vi "ard2.vi"() -> ()   [LabVIEW 2020]
uses:
  <vilib>/Instr/_visa.llb/VISA Configure Serial Port (Instr).vi
panel:
  in  "string":string
  out "concatenated string 2":string
  in  "Boolean 2":bool
  in  "VISA resource name":refnum<visa-resource-name>
  in  "Boolean":bool
  in  "stop":bool
  out "concatenated string":string
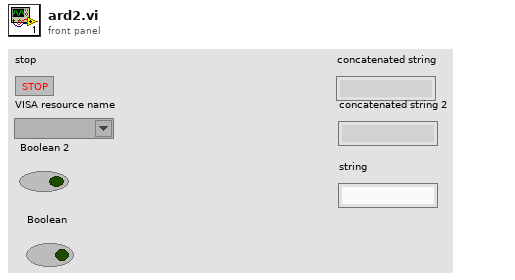
[diagram p1: front panel]
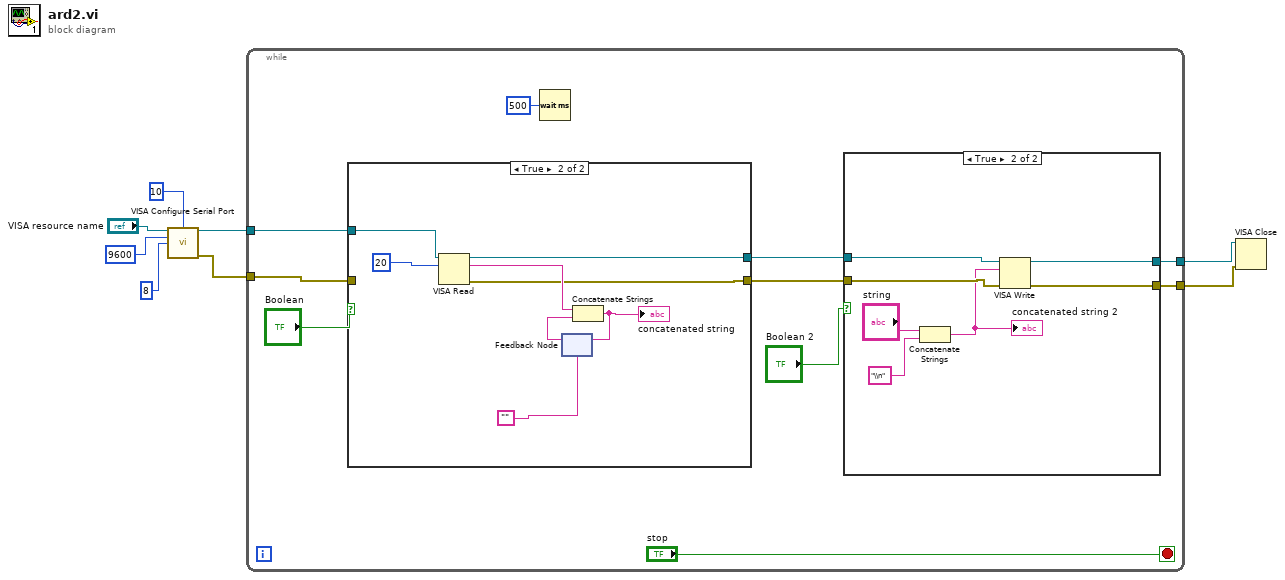
[diagram p0: block diagram]
diagram:
  n1 = call-poly "VISA Configure Serial Port"("VISA resource name"="VISA resource name", "termination char\n(0xA = '\\n' = LF)"=u8 10 ("termination char\n(0xA = '\\n' = LF)"), "baud rate (9600)"=u32 9600, "data bits (8)"=u16 8) -> ("VISA resource name out"=w8:refnum<visa-resource-name>, "error out"=w7:errorcluster)  [unwired: 10 in]
  n2 = while {
    tunnel: w8 -> [w17]
    tunnel: w7 -> [w16]
    tunnel: [w10] -> w2
    tunnel: [w9] -> w1
    stop <- "stop" stop-if-true
    n3 = case shown="True" "Boolean" {
      tunnel: [w28 w31] -> w13
      tunnel: [w29 w33] -> w12
      tunnel: w17 -> [w29 w32]
      tunnel: w16 -> [w28 _]
      frame False {
      }
      frame True {
        n4 = VISA Read(VISA resource name=w32, byte count=u32 20) -> (VISA resource name out=w33:refnum<visa-resource-name>, read buffer=w36:string, error out=w31:errorcluster)  [unwired: 1 in, 1 out]
        n5 = feedback #1("") -> (w34:string)
        n6 = Concatenate Strings(w36, w34) -> (w35:string)
        "concatenated string" <- w35
        n7 = feedback-in #1(w35) -> ()
      }
    }
    n8 = Wait (ms)(milliseconds to wait=u32 500) -> ()  [unwired: 1 out]
    n9 = case shown="True" "Boolean 2" {
      tunnel: w13 -> [w19 w26]
      tunnel: w12 -> [w20 w27]
      tunnel: [w20 w22] -> w10
      tunnel: [w19 w21] -> w9
      frame False {
      }
      frame True {
        n10 = Concatenate Strings("string", "\\n" ("string")) -> (w25:string)
        "concatenated string 2" <- w25
        n11 = VISA Write(VISA resource name=w27, write buffer=w25, error in (no error)=w26) -> (VISA resource name out=w22:refnum<visa-resource-name>, error out=w21:errorcluster)  [unwired: 1 out]
      }
    }
  }
  n12 = VISA Close(VISA resource name=w2, error in (no error)=w1) -> ()  [unwired: 1 out]
